vi "SignalGenerator.vi"() -> ()   [LabVIEW 2015]
panel:
  in  "stop":bool
  out "error in":errorcluster
  out "error out":errorcluster
  in  "Amplitude":i32
  in  "Frequency":i32=10
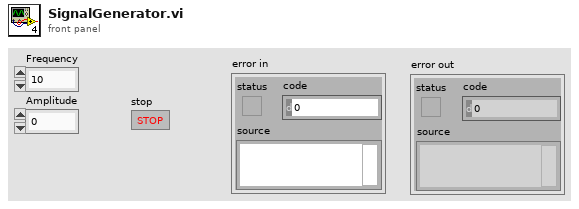
[diagram p1: front panel]
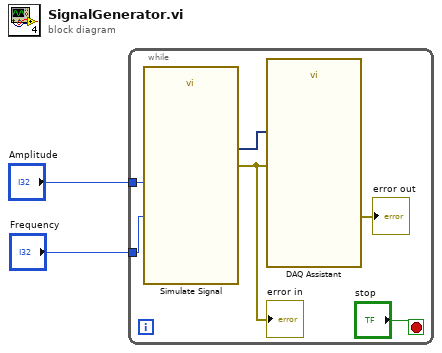
[diagram p0: block diagram]
diagram:
  n1 = while {
    tunnel: "Frequency" -> [w7]
    tunnel: "Amplitude" -> [w6]
    stop <- "stop" stop-if-true
    n2 = call "Simulate Signal"("Frequency"=w7, "Amplitude"=w6) -> ("Sine"=w8:dynamicdata, "error out"=w4:errorcluster)  [unwired: 12 in]
    "error in" <- w4
    n3 = call "DAQ Assistant"("data"=w8, "error in"=w4) -> ("error out"=→"error out":errorcluster)  [unwired: 15 in, 2 out]
  }
